vi "Hardware-HHSetup-Host.vi"() -> ()   [LabVIEW 2016]
uses:
  <vilib>/Powertrain Controls/Device Drivers/DCM/HH/RT/Setup.ctl
  <vilib>/Powertrain Controls/Device Drivers/DCM/HH/FPGA/Mode.ctl
  <vilib>/Powertrain Controls/Device Drivers/DCM/Rev0/FPGA/Digital Channel.ctl
  <vilib>/Powertrain Controls/Device Drivers/DCM/HH/RT/Angle Control.ctl
  Shared/Typedefs/HH-Config-Array.ctl
  <vilib>/Powertrain Controls/Device Drivers/DCM/HH/RT/Mode.ctl
  <vilib>/Powertrain Controls/Device Drivers/DCM/HH/RT/ISeq.ctl
  <vilib>/addons/Software Calibration Management/XControls/SubHost.xctl
  <vilib>/Powertrain Controls/Device Drivers/DCM/HH/FPGA/DCM - FPGA - HH.lvlib
  <vilib>/Powertrain Controls/Device Drivers/DCM/HH/RT/DCM - RT - HH.lvlib
  <vilib>/Powertrain Controls/Device Drivers/DCM/Rev0/FPGA/DCM - FPGA.lvlib
  Shared/DSI-Shared.lvlib
panel:
  in  "_Hidden":enum32{"Page 1"}(tab)
  in  "Config":T1=[{"Mode"=enum."Off", "IO Lock State"=FALSE, "Phase 1 FP"=FALSE, "Fault Clear"=FALSE, "ISeq"=[{"Upper [A]"=0.0, "Lower [A]"=0.0, "Duration [s]"=0.0}, {"Upper [A]"=0.0, "Lower [A]"=0.0, "Duration [s]"=0.0}, {"Upper [A]"=0.0, "Lower [A]"=0.0, "Duration [s]"=0.0}, {"Upper [A]"=0.0, "Lower [A]"=0.0, "Duration [s]"=0.0}]}, {"Mode"=enum."Off", "IO Lock State"=FALSE, "Phase 1 FP"=FALSE, "Fault Clear"=FALSE, "ISeq"=[{"Upper [A]"=0.0, "Lower [A]"=0.0, "Duration [s]"=0.0}, {"Upper [A]"=0.0, "Lower [A]"=0.0, "Duration [s]"=0.0}, {"Upper [A]"=0.0, "Lower [A]"=0.0, "Duration [s]"=0.0}, {"Upper [A]"=0.0, "Lower [A]"=0.0, "Duration [s]"=0.0}]}, {"Mode"=enum."Off", "IO Lock State"=FALSE, "Phase 1 FP"=FALSE, "Fault Clear"=FALSE, "ISeq"=[{"Upper [A]"=0.0, "Lower [A]"=0.0, "Duration [s]"=0.0}, {"Upper [A]"=0.0, "Lower [A]"=0.0, "Duration [s]"=0.0}, {"Upper [A]"=0.0, "Lower [A]"=0.0, "Duration [s]"=0.0}, {"Upper [A]"=0.0, "Lower [A]"=0.0, "Duration [s]"=0.0}]}, {"Mode"=enum."Off", "IO Lock State"=FALSE, "Phase 1 FP"=FALSE, "Fault Clear"=FALSE, "ISeq"=[{"Upper [A]"=0.0, "Lower [A]"=0.0, "Duration [s]"=0.0}, {"Upper [A]"=0.0, "Lower [A]"=0.0, "Duration [s]"=0.0}, {"Upper [A]"=0.0, "Lower [A]"=0.0, "Duration [s]"=0.0}, {"Upper [A]"=0.0, "Lower [A]"=0.0, "Duration [s]"=0.0}]}, {"Mode"=enum."Off", "IO Lock State"=FALSE, "Phase 1 FP"=FALSE, "Fault Clear"=FALSE, "ISeq"=[{"Upper [A]"=0.0, "Lower [A]"=0.0, "Duration [s]"=0.0}, {"Upper [A]"=0.0, "Lower [A]"=0.0, "Duration [s]"=0.0}, {"Upper [A]"=0.0, "Lower [A]"=0.0, "Duration [s]"=0.0}, {"Upper [A]"=0.0, "Lower [A]"=0.0, "Duration [s]"=0.0}]}, {"Mode"=enum."Off", "IO Lock State"=FALSE, "Phase 1 FP"=FALSE, "Fault Clear"=FALSE, "ISeq"=[{"Upper [A]"=0.0, "Lower [A]"=0.0, "Duration [s]"=0.0}, {"Upper [A]"=0.0, "Lower [A]"=0.0, "Duration [s]"=0.0}, {"Upper [A]"=0.0, "Lower [A]"=0.0, "Duration [s]"=0.0}, {"Upper [A]"=0.0, "Lower [A]"=0.0, "Duration [s]"=0.0}]}, {"Mode"=enum."Off", "IO Lock State"=FALSE, "Phase 1 FP"=FALSE, "Fault Clear"=FALSE, "ISeq"=[{"Upper [A]"=0.0, "Lower [A]"=0.0, "Duration [s]"=0.0}, {"Upper [A]"=0.0, "Lower [A]"=0.0, "Duration [s]"=0.0}, {"Upper [A]"=0.0, "Lower [A]"=0.0, "Duration [s]"=0.0}, {"Upper [A]"=0.0, "Lower [A]"=0.0, "Duration [s]"=0.0}]}, {"Mode"=enum."Off", "IO Lock State"=FALSE, "Phase 1 FP"=FALSE, "Fault Clear"=FALSE, "ISeq"=[{"Upper [A]"=0.0, "Lower [A]"=0.0, "Duration [s]"=0.0}, {"Upper [A]"=0.0, "Lower [A]"=0.0, "Duration [s]"=0.0}, {"Upper [A]"=0.0, "Lower [A]"=0.0, "Duration [s]"=0.0}, {"Upper [A]"=0.0, "Lower [A]"=0.0, "Duration [s]"=0.0}]}, {"Mode"=enum."Off", "IO Lock State"=FALSE, "Phase 1 FP"=FALSE, "Fault Clear"=FALSE, "ISeq"=[{"Upper [A]"=0.0, "Lower [A]"=0.0, "Duration [s]"=0.0}, {"Upper [A]"=0.0, "Lower [A]"=0.0, "Duration [s]"=0.0}, {"Upper [A]"=0.0, "Lower [A]"=0.0, "Duration [s]"=0.0}, {"Upper [A]"=0.0, "Lower [A]"=0.0, "Duration [s]"=0.0}]}, {"Mode"=enum."Off", "IO Lock State"=FALSE, "Phase 1 FP"=FALSE, "Fault Clear"=FALSE, "ISeq"=[{"Upper [A]"=0.0, "Lower [A]"=0.0, "Duration [s]"=0.0}, {"Upper [A]"=0.0, "Lower [A]"=0.0, "Duration [s]"=0.0}, {"Upper [A]"=0.0, "Lower [A]"=0.0, "Duration [s]"=0.0}, {"Upper [A]"=0.0, "Lower [A]"=0.0, "Duration [s]"=0.0}]}, {"Mode"=enum."Off", "IO Lock State"=FALSE, "Phase 1 FP"=FALSE, "Fault Clear"=FALSE, "ISeq"=[{"Upper [A]"=0.0, "Lower [A]"=0.0, "Duration [s]"=0.0}, {"Upper [A]"=0.0, "Lower [A]"=0.0, "Duration [s]"=0.0}, {"Upper [A]"=0.0, "Lower [A]"=0.0, "Duration [s]"=0.0}, {"Upper [A]"=0.0, "Lower [A]"=0.0, "Duration [s]"=0.0}]}, {"Mode"=enum."Off", "IO Lock State"=FALSE, "Phase 1 FP"=FALSE, "Fault Clear"=FALSE, "ISeq"=[{"Upper [A]"=0.0, "Lower [A]"=0.0, "Duration [s]"=0.0}, {"Upper [A]"=0.0, "Lower [A]"=0.0, "Duration [s]"=0.0}, {"Upper [A]"=0.0, "Lower [A]"=0.0, "Duration [s]"=0.0}, {"Upper [A]"=0.0, "Lower [A]"=0.0, "Duration [s]"=0.0}]}] {"ISeq"."Duration [s]" min=0 max=26 format="%#_3p"; "ISeq"."Lower [A]" min=0 max=8 format="%#_3p"; "ISeq"."Upper [A]" min=0 max=8 format="%#_3p"}
  in  "Cmd":T4[](array[typedef])=[{"Mode"=enum."Off", "Digital Input"=enum."Unused", "Polarity"=FALSE, "Frequency [Hz]"=0.0, "Duty Cycle [%]"=0.0, "TDC Offset [CAD]"=0.0, "Window Start [DBTDC]"=0.0, "Window End [DBTDC]"=0.0, "Angles"=[{"Enable"=FALSE, "Location [DBTDC]"=0.0, "Duration [s]"=0.0}, {"Enable"=FALSE, "Location [DBTDC]"=0.0, "Duration [s]"=0.0}, {"Enable"=FALSE, "Location [DBTDC]"=0.0, "Duration [s]"=0.0}, {"Enable"=FALSE, "Location [DBTDC]"=0.0, "Duration [s]"=0.0}], "Skip Fire"=FALSE, "Skip Fire Index"=0}, {"Mode"=enum."Off", "Digital Input"=enum."Unused", "Polarity"=FALSE, "Frequency [Hz]"=0.0, "Duty Cycle [%]"=0.0, "TDC Offset [CAD]"=0.0, "Window Start [DBTDC]"=0.0, "Window End [DBTDC]"=0.0, "Angles"=[{"Enable"=FALSE, "Location [DBTDC]"=0.0, "Duration [s]"=0.0}, {"Enable"=FALSE, "Location [DBTDC]"=0.0, "Duration [s]"=0.0}, {"Enable"=FALSE, "Location [DBTDC]"=0.0, "Duration [s]"=0.0}, {"Enable"=FALSE, "Location [DBTDC]"=0.0, "Duration [s]"=0.0}], "Skip Fire"=FALSE, "Skip Fire Index"=0}, {"Mode"=enum."Off", "Digital Input"=enum."Unused", "Polarity"=FALSE, "Frequency [Hz]"=0.0, "Duty Cycle [%]"=0.0, "TDC Offset [CAD]"=0.0, "Window Start [DBTDC]"=0.0, "Window End [DBTDC]"=0.0, "Angles"=[{"Enable"=FALSE, "Location [DBTDC]"=0.0, "Duration [s]"=0.0}, {"Enable"=FALSE, "Location [DBTDC]"=0.0, "Duration [s]"=0.0}, {"Enable"=FALSE, "Location [DBTDC]"=0.0, "Duration [s]"=0.0}, {"Enable"=FALSE, "Location [DBTDC]"=0.0, "Duration [s]"=0.0}], "Skip Fire"=FALSE, "Skip Fire Index"=0}, {"Mode"=enum."Off", "Digital Input"=enum."Unused", "Polarity"=FALSE, "Frequency [Hz]"=0.0, "Duty Cycle [%]"=0.0, "TDC Offset [CAD]"=0.0, "Window Start [DBTDC]"=0.0, "Window End [DBTDC]"=0.0, "Angles"=[{"Enable"=FALSE, "Location [DBTDC]"=0.0, "Duration [s]"=0.0}, {"Enable"=FALSE, "Location [DBTDC]"=0.0, "Duration [s]"=0.0}, {"Enable"=FALSE, "Location [DBTDC]"=0.0, "Duration [s]"=0.0}, {"Enable"=FALSE, "Location [DBTDC]"=0.0, "Duration [s]"=0.0}], "Skip Fire"=FALSE, "Skip Fire Index"=0}, {"Mode"=enum."Off", "Digital Input"=enum."Unused", "Polarity"=FALSE, "Frequency [Hz]"=0.0, "Duty Cycle [%]"=0.0, "TDC Offset [CAD]"=0.0, "Window Start [DBTDC]"=0.0, "Window End [DBTDC]"=0.0, "Angles"=[{"Enable"=FALSE, "Location [DBTDC]"=0.0, "Duration [s]"=0.0}, {"Enable"=FALSE, "Location [DBTDC]"=0.0, "Duration [s]"=0.0}, {"Enable"=FALSE, "Location [DBTDC]"=0.0, "Duration [s]"=0.0}, {"Enable"=FALSE, "Location [DBTDC]"=0.0, "Duration [s]"=0.0}], "Skip Fire"=FALSE, "Skip Fire Index"=0}, {"Mode"=enum."Off", "Digital Input"=enum."Unused", "Polarity"=FALSE, "Frequency [Hz]"=0.0, "Duty Cycle [%]"=0.0, "TDC Offset [CAD]"=0.0, "Window Start [DBTDC]"=0.0, "Window End [DBTDC]"=0.0, "Angles"=[{"Enable"=FALSE, "Location [DBTDC]"=0.0, "Duration [s]"=0.0}, {"Enable"=FALSE, "Location [DBTDC]"=0.0, "Duration [s]"=0.0}, {"Enable"=FALSE, "Location [DBTDC]"=0.0, "Duration [s]"=0.0}, {"Enable"=FALSE, "Location [DBTDC]"=0.0, "Duration [s]"=0.0}], "Skip Fire"=FALSE, "Skip Fire Index"=0}, {"Mode"=enum."Off", "Digital Input"=enum."Unused", "Polarity"=FALSE, "Frequency [Hz]"=0.0, "Duty Cycle [%]"=0.0, "TDC Offset [CAD]"=0.0, "Window Start [DBTDC]"=0.0, "Window End [DBTDC]"=0.0, "Angles"=[{"Enable"=FALSE, "Location [DBTDC]"=0.0, "Duration [s]"=0.0}, {"Enable"=FALSE, "Location [DBTDC]"=0.0, "Duration [s]"=0.0}, {"Enable"=FALSE, "Location [DBTDC]"=0.0, "Duration [s]"=0.0}, {"Enable"=FALSE, "Location [DBTDC]"=0.0, "Duration [s]"=0.0}], "Skip Fire"=FALSE, "Skip Fire Index"=0}, {"Mode"=enum."Off", "Digital Input"=enum."Unused", "Polarity"=FALSE, "Frequency [Hz]"=0.0, "Duty Cycle [%]"=0.0, "TDC Offset [CAD]"=0.0, "Window Start [DBTDC]"=0.0, "Window End [DBTDC]"=0.0, "Angles"=[{"Enable"=FALSE, "Location [DBTDC]"=0.0, "Duration [s]"=0.0}, {"Enable"=FALSE, "Location [DBTDC]"=0.0, "Duration [s]"=0.0}, {"Enable"=FALSE, "Location [DBTDC]"=0.0, "Duration [s]"=0.0}, {"Enable"=FALSE, "Location [DBTDC]"=0.0, "Duration [s]"=0.0}], "Skip Fire"=FALSE, "Skip Fire Index"=0}, {"Mode"=enum."Off", "Digital Input"=enum."Unused", "Polarity"=FALSE, "Frequency [Hz]"=0.0, "Duty Cycle [%]"=0.0, "TDC Offset [CAD]"=0.0, "Window Start [DBTDC]"=0.0, "Window End [DBTDC]"=0.0, "Angles"=[{"Enable"=FALSE, "Location [DBTDC]"=0.0, "Duration [s]"=0.0}, {"Enable"=FALSE, "Location [DBTDC]"=0.0, "Duration [s]"=0.0}, {"Enable"=FALSE, "Location [DBTDC]"=0.0, "Duration [s]"=0.0}, {"Enable"=FALSE, "Location [DBTDC]"=0.0, "Duration [s]"=0.0}], "Skip Fire"=FALSE, "Skip Fire Index"=0}, {"Mode"=enum."Off", "Digital Input"=enum."Unused", "Polarity"=FALSE, "Frequency [Hz]"=0.0, "Duty Cycle [%]"=0.0, "TDC Offset [CAD]"=0.0, "Window Start [DBTDC]"=0.0, "Window End [DBTDC]"=0.0, "Angles"=[{"Enable"=FALSE, "Location [DBTDC]"=0.0, "Duration [s]"=0.0}, {"Enable"=FALSE, "Location [DBTDC]"=0.0, "Duration [s]"=0.0}, {"Enable"=FALSE, "Location [DBTDC]"=0.0, "Duration [s]"=0.0}, {"Enable"=FALSE, "Location [DBTDC]"=0.0, "Duration [s]"=0.0}], "Skip Fire"=FALSE, "Skip Fire Index"=0}, {"Mode"=enum."Off", "Digital Input"=enum."Unused", "Polarity"=FALSE, "Frequency [Hz]"=0.0, "Duty Cycle [%]"=0.0, "TDC Offset [CAD]"=0.0, "Window Start [DBTDC]"=0.0, "Window End [DBTDC]"=0.0, "Angles"=[{"Enable"=FALSE, "Location [DBTDC]"=0.0, "Duration [s]"=0.0}, {"Enable"=FALSE, "Location [DBTDC]"=0.0, "Duration [s]"=0.0}, {"Enable"=FALSE, "Location [DBTDC]"=0.0, "Duration [s]"=0.0}, {"Enable"=FALSE, "Location [DBTDC]"=0.0, "Duration [s]"=0.0}], "Skip Fire"=FALSE, "Skip Fire Index"=0}, {"Mode"=enum."Off", "Digital Input"=enum."Unused", "Polarity"=FALSE, "Frequency [Hz]"=0.0, "Duty Cycle [%]"=0.0, "TDC Offset [CAD]"=0.0, "Window Start [DBTDC]"=0.0, "Window End [DBTDC]"=0.0, "Angles"=[{"Enable"=FALSE, "Location [DBTDC]"=0.0, "Duration [s]"=0.0}, {"Enable"=FALSE, "Location [DBTDC]"=0.0, "Duration [s]"=0.0}, {"Enable"=FALSE, "Location [DBTDC]"=0.0, "Duration [s]"=0.0}, {"Enable"=FALSE, "Location [DBTDC]"=0.0, "Duration [s]"=0.0}], "Skip Fire"=FALSE, "Skip Fire Index"=0}] {"Skip Fire Index" max=7; "Angles"."Duration [s]" format="%#_3p"; "Frequency [Hz]" format="%#_3p"}
  in  "_Refresh":bool
  in  "AdaptMode":u32
  in  "ChannelNames":string[](array[string])
  out "_Disabled Configs":i32[](array[numeric])
  in  "Scope":T8(xcontrol)
  in  "_Config Tab":enum32{"Page 1"}(tab)
  in  "_Cmd Tab":enum32{"Page 1"}(tab)
  in  "_Icon tabs":enum32{"Off", "Lo", "Hi", "PFI", "FullH"}(tab)
  in  "Status":T8(xcontrol)
  in  "_AdaptMode":bool caption="Adapt Mode"
  in  "_Channel Name":string caption="Channel Name"
  in  "_Command Element":T4={"Mode"=enum."Off", "Digital Input"=enum."Unused", "Polarity"=FALSE, "Frequency [Hz]"=0.0, "Duty Cycle [%]"=0.0, "TDC Offset [CAD]"=0.0, "Window Start [DBTDC]"=0.0, "Window End [DBTDC]"=0.0, "Angles"=[{"Enable"=FALSE, "Location [DBTDC]"=0.0, "Duration [s]"=0.0}, {"Enable"=FALSE, "Location [DBTDC]"=0.0, "Duration [s]"=0.0}, {"Enable"=FALSE, "Location [DBTDC]"=0.0, "Duration [s]"=0.0}, {"Enable"=FALSE, "Location [DBTDC]"=0.0, "Duration [s]"=0.0}], "Skip Fire"=FALSE, "Skip Fire Index"=0} caption="Command Setup" {"Skip Fire Index" max=7; "Angles"."Duration [s]" format="%#_3p"; "Frequency [Hz]" format="%#_3p"}
  in  "_Config Element":T9={"Mode"=enum."Off", "IO Lock State"=FALSE, "Phase 1 FP"=FALSE, "Fault Clear"=FALSE, "ISeq"=[{"Upper [A]"=0.0, "Lower [A]"=0.0, "Duration [s]"=0.0}, {"Upper [A]"=0.0, "Lower [A]"=0.0, "Duration [s]"=0.0}, {"Upper [A]"=0.0, "Lower [A]"=0.0, "Duration [s]"=0.0}, {"Upper [A]"=0.0, "Lower [A]"=0.0, "Duration [s]"=0.0}]} caption="Channel Configuration" {"ISeq"."Duration [s]" min=0 max=26 format="%#_3p"; "ISeq"."Lower [A]" min=0 max=8 format="%#_3p"; "ISeq"."Upper [A]" min=0 max=8 format="%#_3p"}
  in  "_HH Channels":i32[](listbox) caption="Half-H Channel Summary"
  # "Half-H Drive Setup & Control"
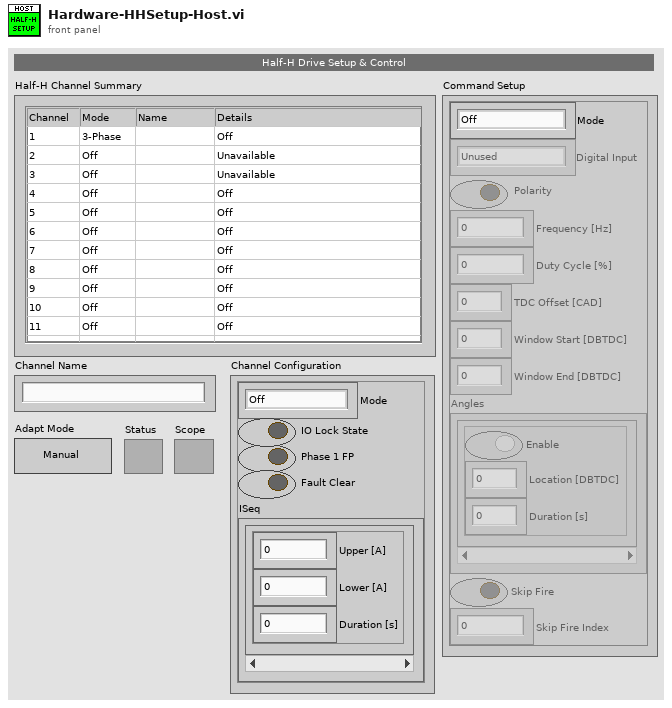
[diagram p1: front panel]
types:
  T1 = typedef "DSI-Shared.lvlib/HH-Config-Array.ctl" = cluster{"Mode":T2, "IO Lock State":bool, "Phase 1 FP":bool, "Fault Clear":bool, "ISeq":T3[]}[]
  T2 = typedef "DCM - RT - HH.lvlib/Mode.ctl" = enum16{"Off", "Lowside", "Highside", "PFI", "Full H", "3-Phase"}
  T3 = typedef "DCM - RT - HH.lvlib/ISeq.ctl" = cluster{"Upper [A]":sgl, "Lower [A]":sgl, "Duration [s]":sgl}
  T4 = typedef "DCM - RT - HH.lvlib/Setup.ctl" = cluster{"Mode":T5, "Digital Input":T6, "Polarity":bool, "Frequency [Hz]":sgl, "Duty Cycle [%]":sgl, "TDC Offset [CAD]":sgl, "Window Start [DBTDC]":sgl, "Window End [DBTDC]":sgl, "Angles":T7[], "Skip Fire":bool, "Skip Fire Index":u8}
  T5 = typedef "DCM - FPGA - HH.lvlib/Mode.ctl" = enum8{"Off", "Direct", "Pulse Width Modulation", "Engine Position Tracking"}
  T6 = typedef "DCM - FPGA.lvlib/Digital Channel.ctl" = enum8{"Unused", "User OS", "Diff IO 1", "Diff IO 2", "Diff IO 3", "Diff IO 4", "Diff IO 5", "Diff IO 6", "Diff IO 7", "Diff IO 8", "Aux 1", "Aux 2", "Aux 3", "Aux 4", "Aux 5", "Aux 6", "Aux 7", "Aux 8", "Aux 9", "Aux 10", "Aux 11", "Aux 12", "Aux 13", "Aux 14", "Aux 15", "Aux 16"}
  T7 = typedef "DCM - RT - HH.lvlib/Angle Control.ctl" = cluster{"Enable":bool, "Location [DBTDC]":sgl, "Duration [s]":sgl}
  T8 = cluster{"Name":string, "Host VI":path, "Pairing File":path, "Display Name":string}
  T9 = cluster{"Mode":T2, "IO Lock State":bool, "Phase 1 FP":bool, "Fault Clear":bool, "ISeq":T3[]}
  T10 = enum8{"Enabled", "Disabled", "Disabled and Grayed Out"}
  T11 = typedef "DCM - RT - HH.lvlib/Config.ctl" = cluster{"Mode":T2, "IO Lock State":bool, "Phase 1 FP":bool, "Fault Clear":bool, "ISeq":T3[]}
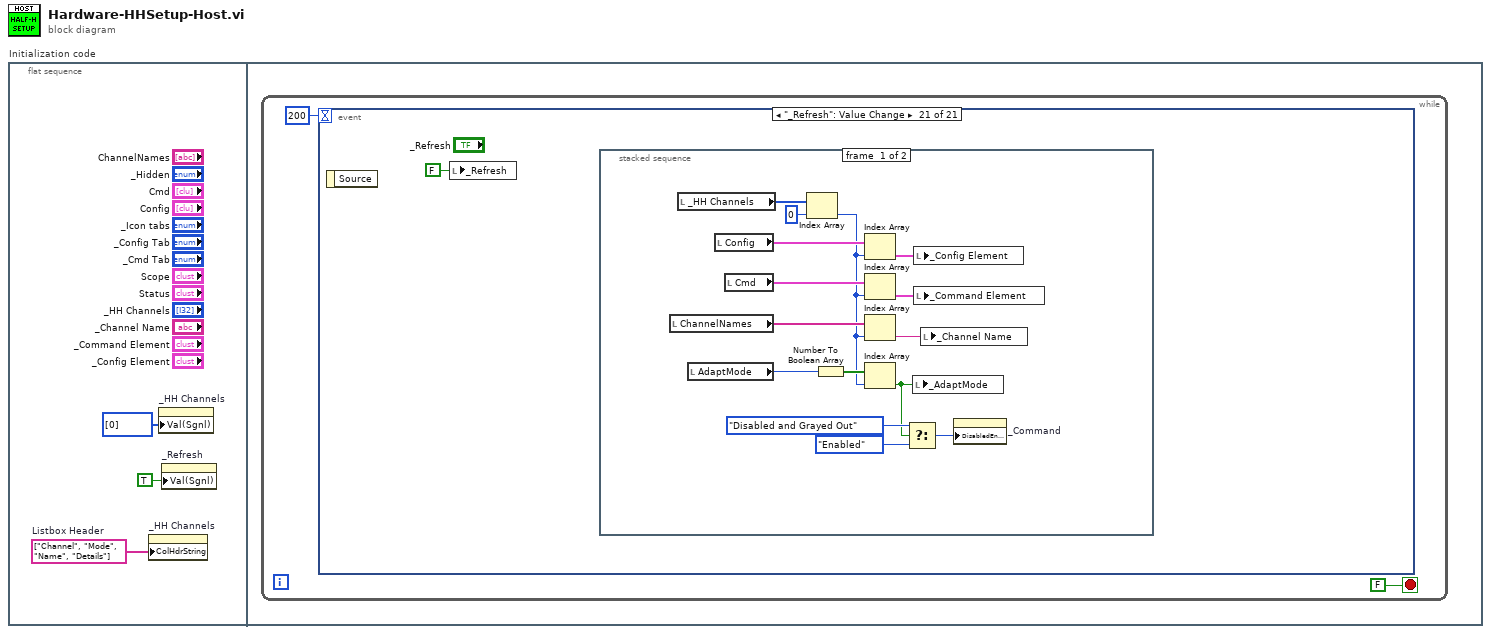
[diagram p0: block diagram]
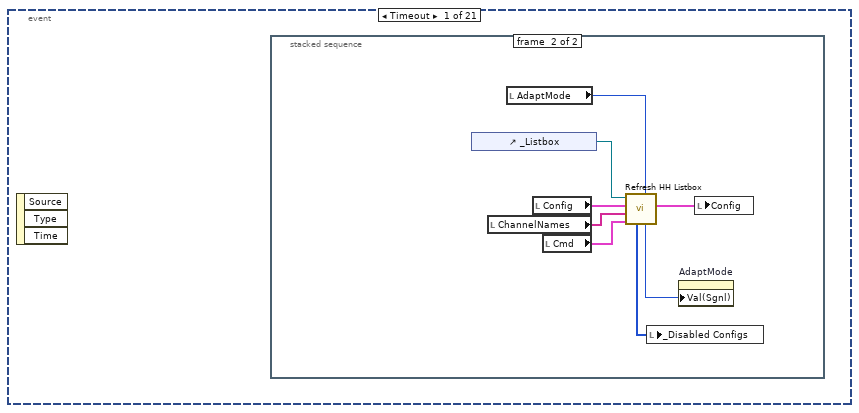
[diagram p2: hidden frame]
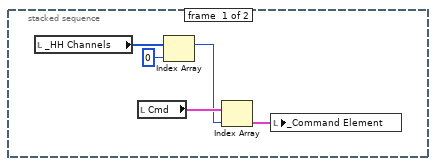
[diagram p3: hidden frame]
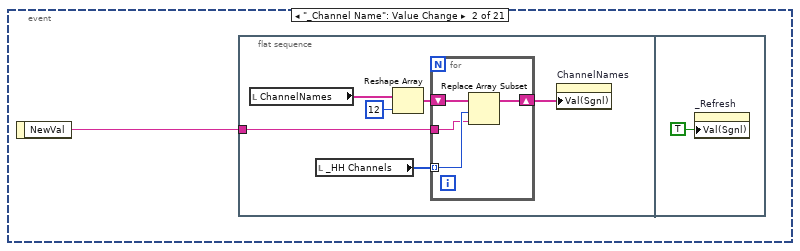
[diagram p4: hidden frame]
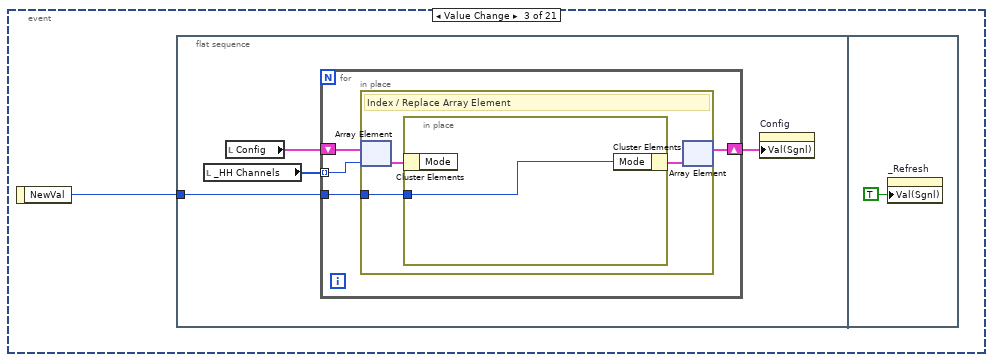
[diagram p5: hidden frame]
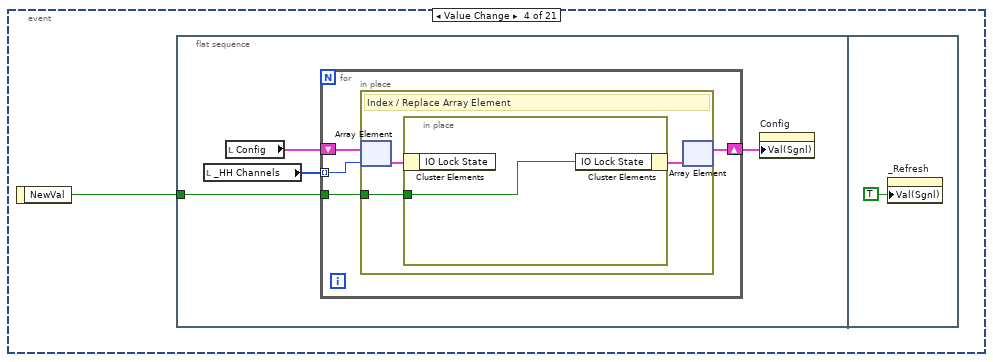
[diagram p6: hidden frame]
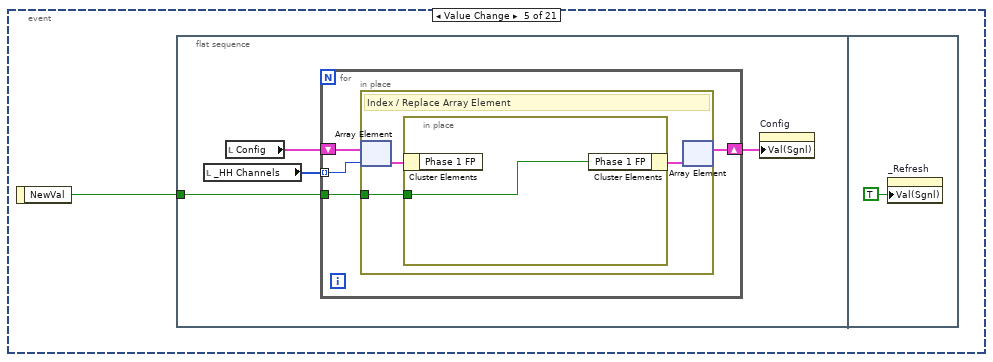
[diagram p7: hidden frame]
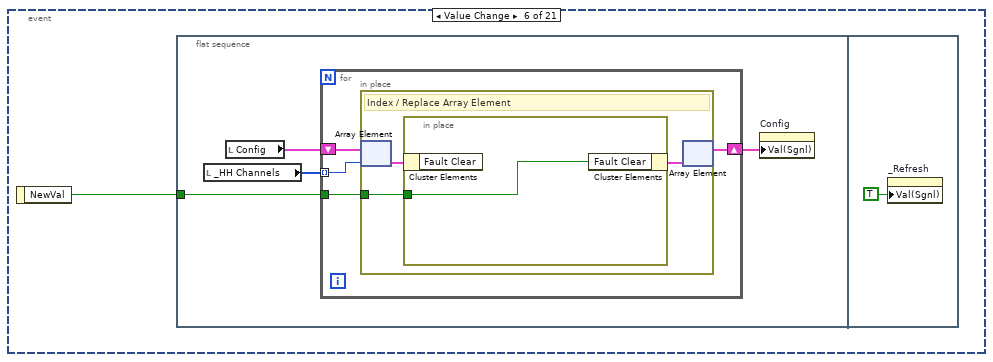
[diagram p8: hidden frame]
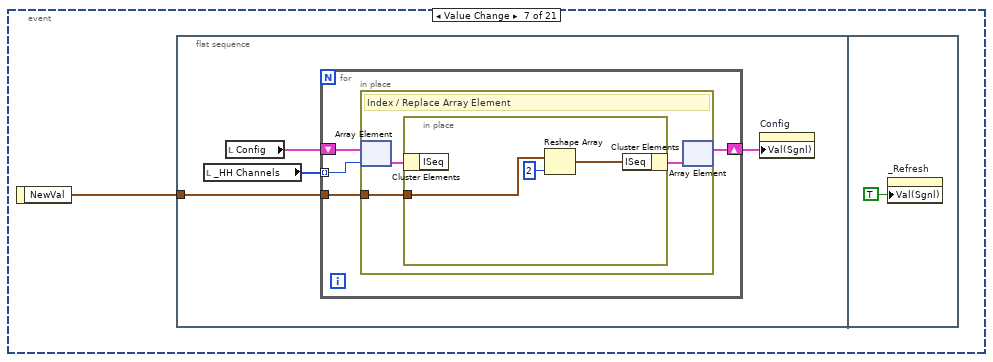
[diagram p9: hidden frame]
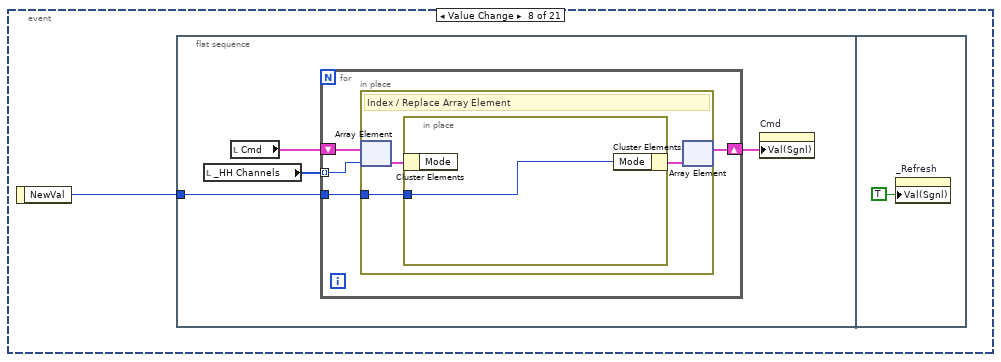
[diagram p10: hidden frame]
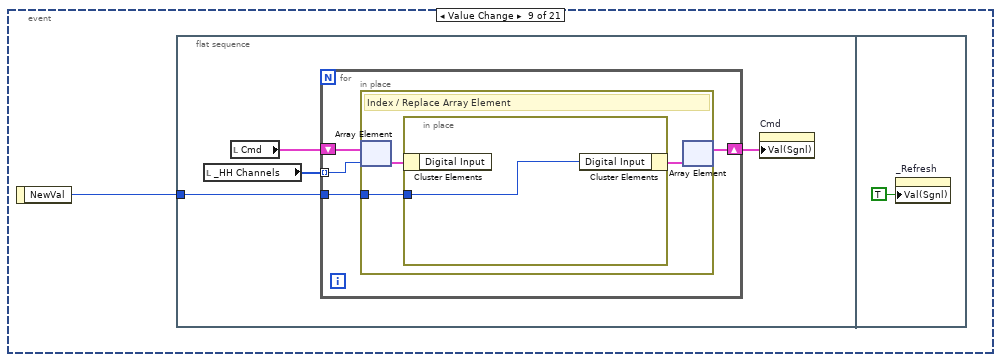
[diagram p11: hidden frame]
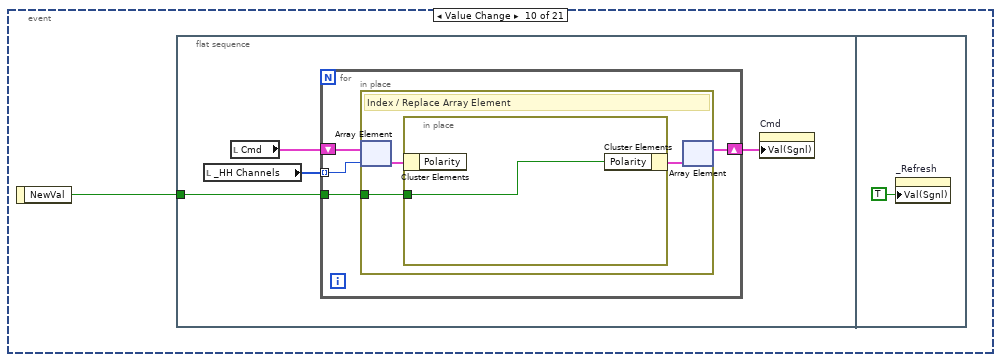
[diagram p12: hidden frame]
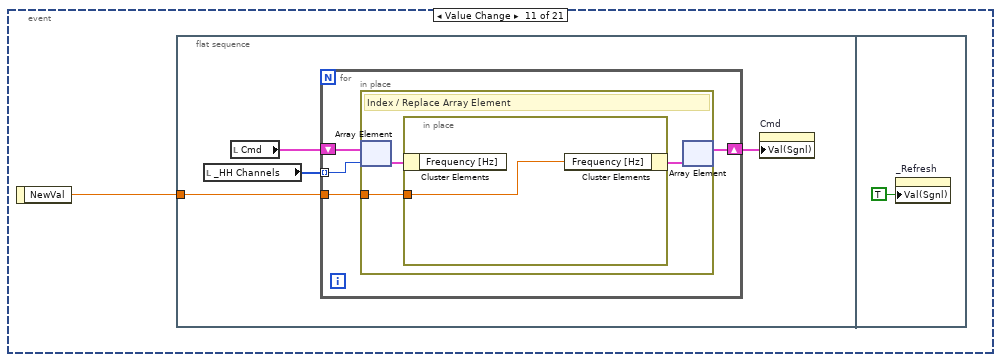
[diagram p13: hidden frame]
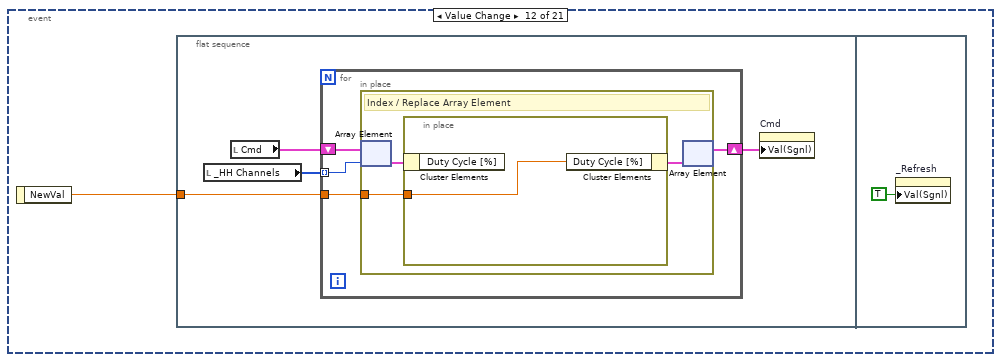
[diagram p14: hidden frame]
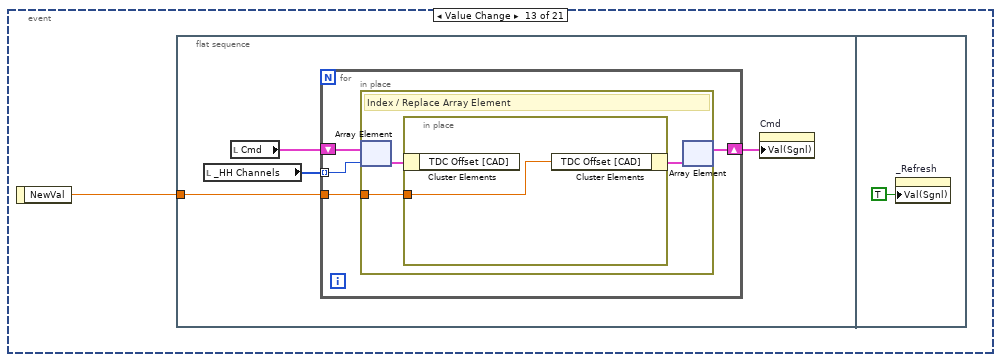
[diagram p15: hidden frame]
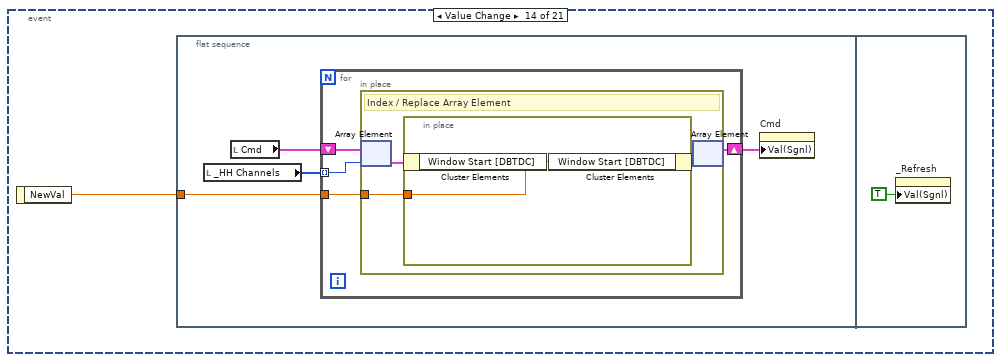
[diagram p16: hidden frame]
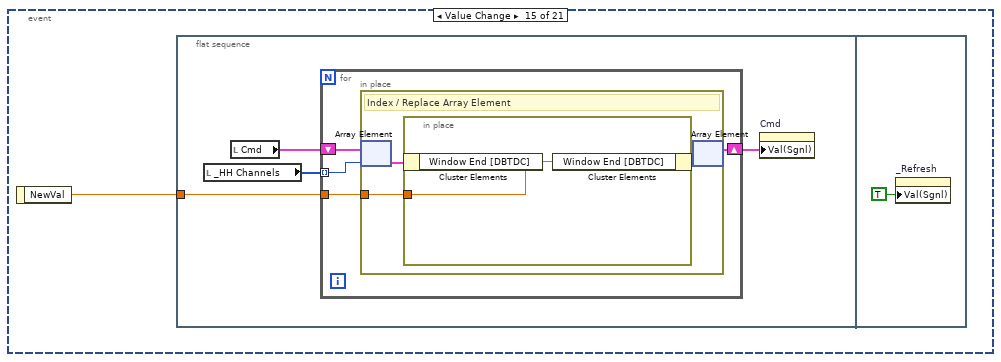
[diagram p17: hidden frame]
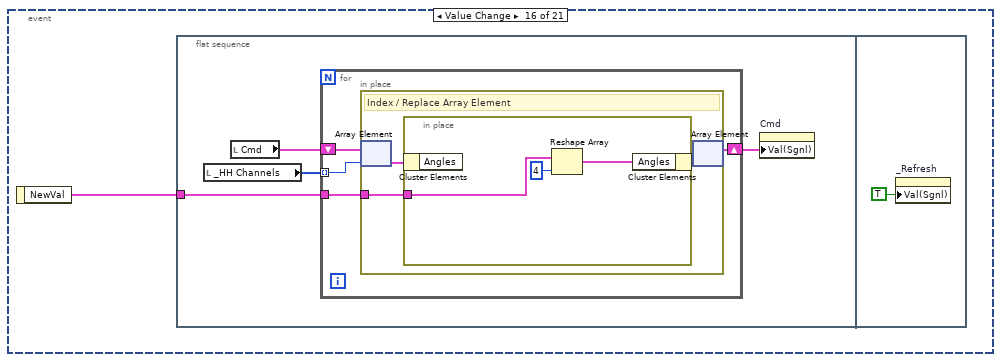
[diagram p18: hidden frame]
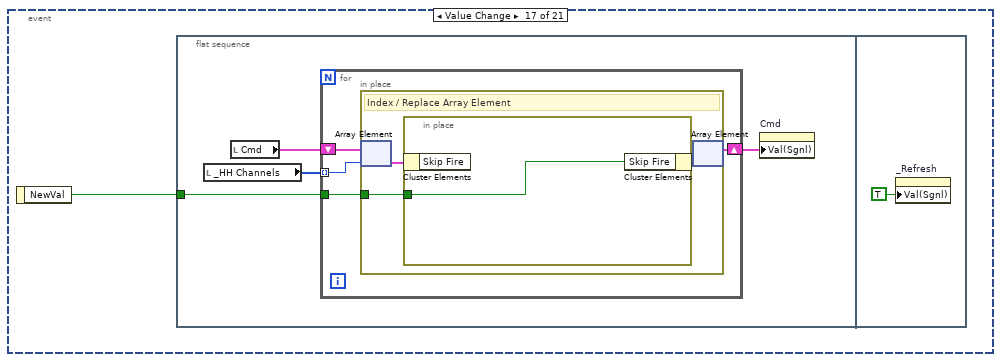
[diagram p19: hidden frame]
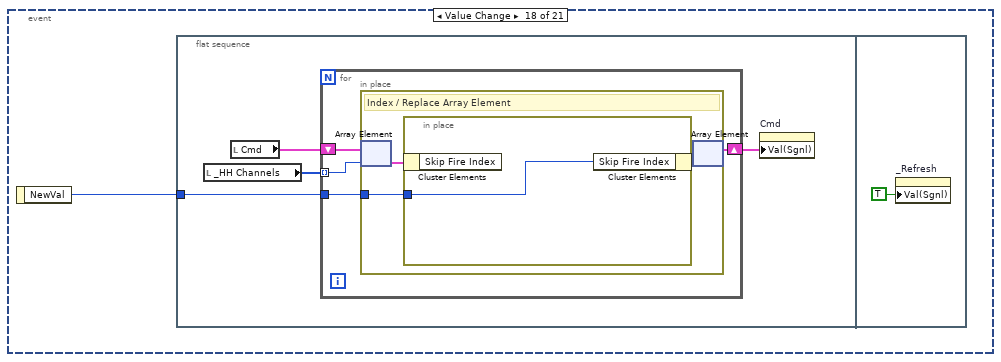
[diagram p20: hidden frame]
diagram:
  n1 = flat-sequence "Initialization code" {
    frame #0 {
      w1 = string[] ["Channel", "Mode", "Name", "Details"]  # Listbox Header
      n2 = property on="_HH Channels" class="MCListbox (strict)"("ColHdrString"=w1) -> ()  [unwired: 2 in, 2 out]
      n3 = property on="_HH Channels" class="MCListbox (strict)"("Val(Sgnl)"=i32[] [0] ("Value (Signaling)")) -> ()  [unwired: 2 in, 2 out]
      n4 = property on="_Refresh" class="Bool (strict)"("Val(Sgnl)"=TRUE ("Value (Signaling)")) -> ()  [unwired: 2 in, 2 out]
    }
    frame #1 {
      n5 = while {
        stop <- FALSE stop-if-true
        n6 = event shown="[20] \"_Refresh\": Value Change" {
          selector: _ -> [_ _ _ _ _ _ _ _ _ _ _ _ _ _ _ _ _ _ _ _ _]
          dyn-events: _ -> [_ _ _ _ _ _ _ _ _ _ _ _ _ _ _ _ _ _ _ _ _]
          timeout: 200 -> [_ _ _ _ _ _ _ _ _ _ _ _ _ _ _ _ _ _ _ _ _]
          event Timeout {
            n7 = event-data() -> ()  [unwired: 4 out]
            n8 = stacked-sequence {
              frame #0 {
                n9 = local read "_HH Channels"() -> (w10:i32[])
                n10 = local read "Cmd"() -> (w9:T4[])
                n11 = Index Array(array=w10, index=0) -> (element=w8:i32)
                n12 = Index Array(array=w9, index=w8) -> (element=w6:T4)
                n13 = local write "_Command Element"(w6) -> ()
              }
              frame #1 {
                n14 = control-ref of="_Listbox"() -> (w13:refnum<vi>)
                n15 = local read "ChannelNames"() -> (w11:string[])
                n16 = local read "AdaptMode"() -> (w16:u32)
                n17 = local read "Config"() -> (w18:T1)
                n18 = local read "Cmd"() -> (w17:T4[])
                n19 = call "Refresh HH Listbox.vi"("AdaptMode"=w16, "Command"=w17, "Names"=w11, "Config"=w18, "_Listbox"=w13) -> ("Config out"=w14:T11[], "AdaptMode"=w15:u32, "Disabled Configs"=w12:i32[])  [unwired: 3 in, 1 out]
                n20 = local write "_Disabled Configs"(w12) -> ()
                n21 = property on="AdaptMode" class="DigNum (strict)"("Val(Sgnl)"=w15) -> ()  [unwired: 2 in, 2 out]
                n22 = local write "Config"(w14) -> ()
              }
            }
          }
          event "_Channel Name": Value Change {
            n23 = event-data() -> ("NewVal"=w19:string)  [unwired: 1 out]
            n24 = flat-sequence {
              tunnel: w19 -> [w22]
              frame #0 {
                n25 = local read "ChannelNames"() -> (w21:string[])
                n26 = local read "_HH Channels"() -> (w25:i32[])
                n27 = Reshape Array(w21, 12 ("dimension size")) -> (w23:string[])
                n28 = for {
                  tunnel: w25 -> [w27] mode=indexing
                  shift-right: [w28] -> w20
                  shift-left: w23 -> [w29]
                  tunnel: w22 -> [w26]
                  n29 = Replace Array Subset(array=w29, new element=w26, index=w27) -> (w28:string[])
                }
                n30 = property on="ChannelNames" class="Arr (strict)"("Val(Sgnl)"=w20) -> ()  [unwired: 2 in, 2 out]
              }
              frame #1 {
                n31 = property on="_Refresh" class="Bool (strict)"("Val(Sgnl)"=TRUE ("Value (Signaling)")) -> ()  [unwired: 2 in, 2 out]
              }
            }
          }
          event Value Change {
            n32 = event-data() -> ("NewVal"=w31:T2)  [unwired: 1 out]
            n33 = flat-sequence {
              tunnel: w31 -> [w34]
              frame #0 {
                n34 = local read "_HH Channels"() -> (w35:i32[])
                n35 = local read "Config"() -> (w33:T1)
                n36 = for {
                  tunnel: w35 -> [w38] mode=indexing
                  shift-right: [w37] -> w32
                  shift-left: w33 -> [w39]
                  tunnel: w34 -> [w36]
                  n37 = in-place {
                    in-place-border: w36 -> [w40]
                    # "Index / Replace Array Element"
                    n38 = in-place-array #1(w39, w38) -> (w42:T9)
                    n39 = in-place {
                      in-place-border: w40 -> [w43]
                      n40 = in-place-cluster #2(w42) -> ()  [unwired: 1 out]
                      n41 = in-place-cluster #2("Mode"=w43) -> (w41:T9)
                    }
                    n42 = in-place-array #1(w41) -> (w37:T1)  [unwired: 1 out]
                  }
                }
                n43 = property on="Config" class="Arr (strict)"("Val(Sgnl)"=w32) -> ()  [unwired: 2 in, 2 out]
              }
              frame #1 {
                n44 = property on="_Refresh" class="Bool (strict)"("Val(Sgnl)"=TRUE ("Value (Signaling)")) -> ()  [unwired: 2 in, 2 out]
              }
            }
          }
          event "_Config Element.IO Lock State": Value Change {
            n45 = event-data() -> ("NewVal"=w45:bool)  [unwired: 1 out]
            n46 = flat-sequence {
              tunnel: w45 -> [w48]
              frame #0 {
                n47 = local read "_HH Channels"() -> (w49:i32[])
                n48 = local read "Config"() -> (w47:T1)
                n49 = for {
                  tunnel: w49 -> [w52] mode=indexing
                  shift-right: [w51] -> w46
                  shift-left: w47 -> [w53]
                  tunnel: w48 -> [w50]
                  n50 = in-place {
                    in-place-border: w50 -> [w54]
                    # "Index / Replace Array Element"
                    n51 = in-place-array #3(w53, w52) -> (w56:T9)
                    n52 = in-place {
                      in-place-border: w54 -> [w57]
                      n53 = in-place-cluster #4(w56) -> ()  [unwired: 1 out]
                      n54 = in-place-cluster #4("IO Lock State"=w57) -> (w55:T9)
                    }
                    n55 = in-place-array #3(w55) -> (w51:T1)  [unwired: 1 out]
                  }
                }
                n56 = property on="Config" class="Arr (strict)"("Val(Sgnl)"=w46) -> ()  [unwired: 2 in, 2 out]
              }
              frame #1 {
                n57 = property on="_Refresh" class="Bool (strict)"("Val(Sgnl)"=TRUE ("Value (Signaling)")) -> ()  [unwired: 2 in, 2 out]
              }
            }
          }
          event "_Config Element.Phase 1 FP": Value Change {
            n58 = event-data() -> ("NewVal"=w59:bool)  [unwired: 1 out]
            n59 = flat-sequence {
              tunnel: w59 -> [w62]
              frame #0 {
                n60 = local read "_HH Channels"() -> (w63:i32[])
                n61 = local read "Config"() -> (w61:T1)
                n62 = for {
                  tunnel: w63 -> [w66] mode=indexing
                  shift-right: [w65] -> w60
                  shift-left: w61 -> [w67]
                  tunnel: w62 -> [w64]
                  n63 = in-place {
                    in-place-border: w64 -> [w68]
                    # "Index / Replace Array Element"
                    n64 = in-place-array #5(w67, w66) -> (w70:T9)
                    n65 = in-place {
                      in-place-border: w68 -> [w71]
                      n66 = in-place-cluster #6(w70) -> ()  [unwired: 1 out]
                      n67 = in-place-cluster #6("Phase 1 FP"=w71) -> (w69:T9)
                    }
                    n68 = in-place-array #5(w69) -> (w65:T1)  [unwired: 1 out]
                  }
                }
                n69 = property on="Config" class="Arr (strict)"("Val(Sgnl)"=w60) -> ()  [unwired: 2 in, 2 out]
              }
              frame #1 {
                n70 = property on="_Refresh" class="Bool (strict)"("Val(Sgnl)"=TRUE ("Value (Signaling)")) -> ()  [unwired: 2 in, 2 out]
              }
            }
          }
          event "_Config Element.Fault Clear": Value Change {
            n71 = event-data() -> ("NewVal"=w73:bool)  [unwired: 1 out]
            n72 = flat-sequence {
              tunnel: w73 -> [w76]
              frame #0 {
                n73 = local read "_HH Channels"() -> (w77:i32[])
                n74 = local read "Config"() -> (w75:T1)
                n75 = for {
                  tunnel: w77 -> [w80] mode=indexing
                  shift-right: [w79] -> w74
                  shift-left: w75 -> [w81]
                  tunnel: w76 -> [w78]
                  n76 = in-place {
                    in-place-border: w78 -> [w82]
                    # "Index / Replace Array Element"
                    n77 = in-place-array #7(w81, w80) -> (w84:T9)
                    n78 = in-place {
                      in-place-border: w82 -> [w85]
                      n79 = in-place-cluster #8(w84) -> ()  [unwired: 1 out]
                      n80 = in-place-cluster #8("Fault Clear"=w85) -> (w83:T9)
                    }
                    n81 = in-place-array #7(w83) -> (w79:T1)  [unwired: 1 out]
                  }
                }
                n82 = property on="Config" class="Arr (strict)"("Val(Sgnl)"=w74) -> ()  [unwired: 2 in, 2 out]
              }
              frame #1 {
                n83 = property on="_Refresh" class="Bool (strict)"("Val(Sgnl)"=TRUE ("Value (Signaling)")) -> ()  [unwired: 2 in, 2 out]
              }
            }
          }
          event "_Config Element.ISeq": Value Change {
            n84 = event-data() -> ("NewVal"=w87:T3[])  [unwired: 1 out]
            n85 = flat-sequence {
              tunnel: w87 -> [w90]
              frame #0 {
                n86 = local read "_HH Channels"() -> (w91:i32[])
                n87 = local read "Config"() -> (w89:T1)
                n88 = for {
                  tunnel: w91 -> [w94] mode=indexing
                  shift-right: [w93] -> w88
                  shift-left: w89 -> [w95]
                  tunnel: w90 -> [w92]
                  n89 = in-place {
                    in-place-border: w92 -> [w96]
                    # "Index / Replace Array Element"
                    n90 = in-place-array #9(w95, w94) -> (w98:T9)
                    n91 = in-place {
                      in-place-border: w96 -> [w100]
                      n92 = in-place-cluster #10(w98) -> ()  [unwired: 1 out]
                      n93 = Reshape Array(w100, 2 ("dimension size")) -> (w99:T3[])
                      n94 = in-place-cluster #10("ISeq"=w99) -> (w97:T9)
                    }
                    n95 = in-place-array #9(w97) -> (w93:T1)  [unwired: 1 out]
                  }
                }
                n96 = property on="Config" class="Arr (strict)"("Val(Sgnl)"=w88) -> ()  [unwired: 2 in, 2 out]
              }
              frame #1 {
                n97 = property on="_Refresh" class="Bool (strict)"("Val(Sgnl)"=TRUE ("Value (Signaling)")) -> ()  [unwired: 2 in, 2 out]
              }
            }
          }
          event Value Change {
            n98 = event-data() -> ("NewVal"=w103:T5)  [unwired: 1 out]
            n99 = flat-sequence {
              tunnel: w103 -> [w106]
              frame #0 {
                n100 = local read "_HH Channels"() -> (w107:i32[])
                n101 = local read "Cmd"() -> (w105:T4[])
                n102 = for {
                  tunnel: w107 -> [w110] mode=indexing
                  shift-right: [w109] -> w104
                  shift-left: w105 -> [w111]
                  tunnel: w106 -> [w108]
                  n103 = in-place {
                    in-place-border: w108 -> [w112]
                    # "Index / Replace Array Element"
                    n104 = in-place-array #11(w111, w110) -> (w114:T4)
                    n105 = in-place {
                      in-place-border: w112 -> [w115]
                      n106 = in-place-cluster #12(w114) -> ()  [unwired: 1 out]
                      n107 = in-place-cluster #12("Mode"=w115) -> (w113:T4)
                    }
                    n108 = in-place-array #11(w113) -> (w109:T4[])  [unwired: 1 out]
                  }
                }
                n109 = property on="Cmd" class="Arr (strict)"("Val(Sgnl)"=w104) -> ()  [unwired: 2 in, 2 out]
              }
              frame #1 {
                n110 = property on="_Refresh" class="Bool (strict)"("Val(Sgnl)"=TRUE ("Value (Signaling)")) -> ()  [unwired: 2 in, 2 out]
              }
            }
          }
          event Value Change {
            n111 = event-data() -> ("NewVal"=w117:T6)  [unwired: 1 out]
            n112 = flat-sequence {
              tunnel: w117 -> [w120]
              frame #0 {
                n113 = local read "_HH Channels"() -> (w121:i32[])
                n114 = local read "Cmd"() -> (w119:T4[])
                n115 = for {
                  tunnel: w121 -> [w124] mode=indexing
                  shift-right: [w123] -> w118
                  shift-left: w119 -> [w125]
                  tunnel: w120 -> [w122]
                  n116 = in-place {
                    in-place-border: w122 -> [w126]
                    # "Index / Replace Array Element"
                    n117 = in-place-array #13(w125, w124) -> (w128:T4)
                    n118 = in-place {
                      in-place-border: w126 -> [w129]
                      n119 = in-place-cluster #14(w128) -> ()  [unwired: 1 out]
                      n120 = in-place-cluster #14("Digital Input"=w129) -> (w127:T4)
                    }
                    n121 = in-place-array #13(w127) -> (w123:T4[])  [unwired: 1 out]
                  }
                }
                n122 = property on="Cmd" class="Arr (strict)"("Val(Sgnl)"=w118) -> ()  [unwired: 2 in, 2 out]
              }
              frame #1 {
                n123 = property on="_Refresh" class="Bool (strict)"("Val(Sgnl)"=TRUE ("Value (Signaling)")) -> ()  [unwired: 2 in, 2 out]
              }
            }
          }
          event Value Change {
            n124 = event-data() -> ("NewVal"=w131:bool)  [unwired: 1 out]
            n125 = flat-sequence {
              tunnel: w131 -> [w134]
              frame #0 {
                n126 = local read "_HH Channels"() -> (w135:i32[])
                n127 = local read "Cmd"() -> (w133:T4[])
                n128 = for {
                  tunnel: w135 -> [w138] mode=indexing
                  shift-right: [w137] -> w132
                  shift-left: w133 -> [w139]
                  tunnel: w134 -> [w136]
                  n129 = in-place {
                    in-place-border: w136 -> [w140]
                    # "Index / Replace Array Element"
                    n130 = in-place-array #15(w139, w138) -> (w142:T4)
                    n131 = in-place {
                      in-place-border: w140 -> [w143]
                      n132 = in-place-cluster #16(w142) -> ()  [unwired: 1 out]
                      n133 = in-place-cluster #16("Polarity"=w143) -> (w141:T4)
                    }
                    n134 = in-place-array #15(w141) -> (w137:T4[])  [unwired: 1 out]
                  }
                }
                n135 = property on="Cmd" class="Arr (strict)"("Val(Sgnl)"=w132) -> ()  [unwired: 2 in, 2 out]
              }
              frame #1 {
                n136 = property on="_Refresh" class="Bool (strict)"("Val(Sgnl)"=TRUE ("Value (Signaling)")) -> ()  [unwired: 2 in, 2 out]
              }
            }
          }
          event Value Change {
            n137 = event-data() -> ("NewVal"=w145:sgl)  [unwired: 1 out]
            n138 = flat-sequence {
              tunnel: w145 -> [w148]
              frame #0 {
                n139 = local read "_HH Channels"() -> (w149:i32[])
                n140 = local read "Cmd"() -> (w147:T4[])
                n141 = for {
                  tunnel: w149 -> [w152] mode=indexing
                  shift-right: [w151] -> w146
                  shift-left: w147 -> [w153]
                  tunnel: w148 -> [w150]
                  n142 = in-place {
                    in-place-border: w150 -> [w154]
                    # "Index / Replace Array Element"
                    n143 = in-place-array #17(w153, w152) -> (w156:T4)
                    n144 = in-place {
                      in-place-border: w154 -> [w157]
                      n145 = in-place-cluster #18(w156) -> ()  [unwired: 1 out]
                      n146 = in-place-cluster #18("Frequency [Hz]"=w157) -> (w155:T4)
                    }
                    n147 = in-place-array #17(w155) -> (w151:T4[])  [unwired: 1 out]
                  }
                }
                n148 = property on="Cmd" class="Arr (strict)"("Val(Sgnl)"=w146) -> ()  [unwired: 2 in, 2 out]
              }
              frame #1 {
                n149 = property on="_Refresh" class="Bool (strict)"("Val(Sgnl)"=TRUE ("Value (Signaling)")) -> ()  [unwired: 2 in, 2 out]
              }
            }
          }
          event Value Change {
            n150 = event-data() -> ("NewVal"=w159:sgl)  [unwired: 1 out]
            n151 = flat-sequence {
              tunnel: w159 -> [w162]
              frame #0 {
                n152 = local read "_HH Channels"() -> (w163:i32[])
                n153 = local read "Cmd"() -> (w161:T4[])
                n154 = for {
                  tunnel: w163 -> [w166] mode=indexing
                  shift-right: [w165] -> w160
                  shift-left: w161 -> [w167]
                  tunnel: w162 -> [w164]
                  n155 = in-place {
                    in-place-border: w164 -> [w168]
                    # "Index / Replace Array Element"
                    n156 = in-place-array #19(w167, w166) -> (w170:T4)
                    n157 = in-place {
                      in-place-border: w168 -> [w171]
                      n158 = in-place-cluster #20(w170) -> ()  [unwired: 1 out]
                      n159 = in-place-cluster #20("Duty Cycle [%]"=w171) -> (w169:T4)
                    }
                    n160 = in-place-array #19(w169) -> (w165:T4[])  [unwired: 1 out]
                  }
                }
                n161 = property on="Cmd" class="Arr (strict)"("Val(Sgnl)"=w160) -> ()  [unwired: 2 in, 2 out]
              }
              frame #1 {
                n162 = property on="_Refresh" class="Bool (strict)"("Val(Sgnl)"=TRUE ("Value (Signaling)")) -> ()  [unwired: 2 in, 2 out]
              }
            }
          }
          event Value Change {
            n163 = event-data() -> ("NewVal"=w173:sgl)  [unwired: 1 out]
            n164 = flat-sequence {
              tunnel: w173 -> [w176]
              frame #0 {
                n165 = local read "_HH Channels"() -> (w177:i32[])
                n166 = local read "Cmd"() -> (w175:T4[])
                n167 = for {
                  tunnel: w177 -> [w180] mode=indexing
                  shift-right: [w179] -> w174
                  shift-left: w175 -> [w181]
                  tunnel: w176 -> [w178]
                  n168 = in-place {
                    in-place-border: w178 -> [w182]
                    # "Index / Replace Array Element"
                    n169 = in-place-array #21(w181, w180) -> (w184:T4)
                    n170 = in-place {
                      in-place-border: w182 -> [w185]
                      n171 = in-place-cluster #22(w184) -> ()  [unwired: 1 out]
                      n172 = in-place-cluster #22("TDC Offset [CAD]"=w185) -> (w183:T4)
                    }
                    n173 = in-place-array #21(w183) -> (w179:T4[])  [unwired: 1 out]
                  }
                }
                n174 = property on="Cmd" class="Arr (strict)"("Val(Sgnl)"=w174) -> ()  [unwired: 2 in, 2 out]
              }
              frame #1 {
                n175 = property on="_Refresh" class="Bool (strict)"("Val(Sgnl)"=TRUE ("Value (Signaling)")) -> ()  [unwired: 2 in, 2 out]
              }
            }
          }
          event Value Change {
            n176 = event-data() -> ("NewVal"=w187:sgl)  [unwired: 1 out]
            n177 = flat-sequence {
              tunnel: w187 -> [w190]
              frame #0 {
                n178 = local read "_HH Channels"() -> (w191:i32[])
                n179 = local read "Cmd"() -> (w189:T4[])
                n180 = for {
                  tunnel: w191 -> [w194] mode=indexing
                  shift-right: [w193] -> w188
                  shift-left: w189 -> [w195]
                  tunnel: w190 -> [w192]
                  n181 = in-place {
                    in-place-border: w192 -> [w196]
                    # "Index / Replace Array Element"
                    n182 = in-place-array #23(w195, w194) -> (w198:T4)
                    n183 = in-place {
                      in-place-border: w196 -> [w199]
                      n184 = in-place-cluster #24(w198) -> ()  [unwired: 1 out]
                      n185 = in-place-cluster #24("Window Start [DBTDC]"=w199) -> (w197:T4)
                    }
                    n186 = in-place-array #23(w197) -> (w193:T4[])  [unwired: 1 out]
                  }
                }
                n187 = property on="Cmd" class="Arr (strict)"("Val(Sgnl)"=w188) -> ()  [unwired: 2 in, 2 out]
              }
              frame #1 {
                n188 = property on="_Refresh" class="Bool (strict)"("Val(Sgnl)"=TRUE ("Value (Signaling)")) -> ()  [unwired: 2 in, 2 out]
              }
            }
          }
          event Value Change {
            n189 = event-data() -> ("NewVal"=w201:sgl)  [unwired: 1 out]
            n190 = flat-sequence {
              tunnel: w201 -> [w204]
              frame #0 {
                n191 = local read "_HH Channels"() -> (w205:i32[])
                n192 = local read "Cmd"() -> (w203:T4[])
                n193 = for {
                  tunnel: w205 -> [w208] mode=indexing
                  shift-right: [w207] -> w202
                  shift-left: w203 -> [w209]
                  tunnel: w204 -> [w206]
                  n194 = in-place {
                    in-place-border: w206 -> [w210]
                    # "Index / Replace Array Element"
                    n195 = in-place-array #25(w209, w208) -> (w212:T4)
                    n196 = in-place {
                      in-place-border: w210 -> [w213]
                      n197 = in-place-cluster #26(w212) -> ()  [unwired: 1 out]
                      n198 = in-place-cluster #26("Window End [DBTDC]"=w213) -> (w211:T4)
                    }
                    n199 = in-place-array #25(w211) -> (w207:T4[])  [unwired: 1 out]
                  }
                }
                n200 = property on="Cmd" class="Arr (strict)"("Val(Sgnl)"=w202) -> ()  [unwired: 2 in, 2 out]
              }
              frame #1 {
                n201 = property on="_Refresh" class="Bool (strict)"("Val(Sgnl)"=TRUE ("Value (Signaling)")) -> ()  [unwired: 2 in, 2 out]
              }
            }
          }
          event Value Change {
            n202 = event-data() -> ("NewVal"=w215:T7[])  [unwired: 1 out]
            n203 = flat-sequence {
              tunnel: w215 -> [w218]
              frame #0 {
                n204 = local read "_HH Channels"() -> (w219:i32[])
                n205 = local read "Cmd"() -> (w217:T4[])
                n206 = for {
                  tunnel: w219 -> [w222] mode=indexing
                  shift-right: [w221] -> w216
                  shift-left: w217 -> [w223]
                  tunnel: w218 -> [w220]
                  n207 = in-place {
                    in-place-border: w220 -> [w224]
                    # "Index / Replace Array Element"
                    n208 = in-place-array #27(w223, w222) -> (w226:T4)
                    n209 = in-place {
                      in-place-border: w224 -> [w228]
                      n210 = in-place-cluster #28(w226) -> ()  [unwired: 1 out]
                      n211 = Reshape Array(w228, 4 ("dimension size")) -> (w227:T7[])
                      n212 = in-place-cluster #28("Angles"=w227) -> (w225:T4)
                    }
                    n213 = in-place-array #27(w225) -> (w221:T4[])  [unwired: 1 out]
                  }
                }
                n214 = property on="Cmd" class="Arr (strict)"("Val(Sgnl)"=w216) -> ()  [unwired: 2 in, 2 out]
              }
              frame #1 {
                n215 = property on="_Refresh" class="Bool (strict)"("Val(Sgnl)"=TRUE ("Value (Signaling)")) -> ()  [unwired: 2 in, 2 out]
              }
            }
          }
          event Value Change {
            n216 = event-data() -> ("NewVal"=w231:bool)  [unwired: 1 out]
            n217 = flat-sequence {
              tunnel: w231 -> [w234]
              frame #0 {
                n218 = local read "_HH Channels"() -> (w235:i32[])
                n219 = local read "Cmd"() -> (w233:T4[])
                n220 = for {
                  tunnel: w235 -> [w238] mode=indexing
                  shift-right: [w237] -> w232
                  shift-left: w233 -> [w239]
                  tunnel: w234 -> [w236]
                  n221 = in-place {
                    in-place-border: w236 -> [w240]
                    # "Index / Replace Array Element"
                    n222 = in-place-array #29(w239, w238) -> (w242:T4)
                    n223 = in-place {
                      in-place-border: w240 -> [w243]
                      n224 = in-place-cluster #30(w242) -> ()  [unwired: 1 out]
                      n225 = in-place-cluster #30("Skip Fire"=w243) -> (w241:T4)
                    }
                    n226 = in-place-array #29(w241) -> (w237:T4[])  [unwired: 1 out]
                  }
                }
                n227 = property on="Cmd" class="Arr (strict)"("Val(Sgnl)"=w232) -> ()  [unwired: 2 in, 2 out]
              }
              frame #1 {
                n228 = property on="_Refresh" class="Bool (strict)"("Val(Sgnl)"=TRUE ("Value (Signaling)")) -> ()  [unwired: 2 in, 2 out]
              }
            }
          }
          event Value Change {
            n229 = event-data() -> ("NewVal"=w245:u8)  [unwired: 1 out]
            n230 = flat-sequence {
              tunnel: w245 -> [w248]
              frame #0 {
                n231 = local read "_HH Channels"() -> (w249:i32[])
                n232 = local read "Cmd"() -> (w247:T4[])
                n233 = for {
                  tunnel: w249 -> [w252] mode=indexing
                  shift-right: [w251] -> w246
                  shift-left: w247 -> [w253]
                  tunnel: w248 -> [w250]
                  n234 = in-place {
                    in-place-border: w250 -> [w254]
                    # "Index / Replace Array Element"
                    n235 = in-place-array #31(w253, w252) -> (w256:T4)
                    n236 = in-place {
                      in-place-border: w254 -> [w257]
                      n237 = in-place-cluster #32(w256) -> ()  [unwired: 1 out]
                      n238 = in-place-cluster #32("Skip Fire Index"=w257) -> (w255:T4)
                    }
                    n239 = in-place-array #31(w255) -> (w251:T4[])  [unwired: 1 out]
                  }
                }
                n240 = property on="Cmd" class="Arr (strict)"("Val(Sgnl)"=w246) -> ()  [unwired: 2 in, 2 out]
              }
              frame #1 {
                n241 = property on="_Refresh" class="Bool (strict)"("Val(Sgnl)"=TRUE ("Value (Signaling)")) -> ()  [unwired: 2 in, 2 out]
              }
            }
          }
          event "_AdaptMode": Value Change {
            n242 = event-data() -> ()  [unwired: 7 out]
            n243 = local read "_HH Channels"() -> (w263:i32[])
            n244 = Number To Boolean Array(number="AdaptMode") -> (Boolean array=w261:bool[])
            n245 = for {
              tunnel: "_AdaptMode" -> [w272]
              shift-right: [w270] -> w260
              shift-left: w261 -> [w269]
              tunnel: w263 -> [w271] mode=indexing
              n246 = Replace Array Subset(array=w269, new element=w272, index=w271) -> (w270:bool[])
            }
            n247 = Select(t=T10."Disabled and Grayed Out" ("Disabled"), s="_AdaptMode", f=T10."Enabled" ("Disabled")) -> (s? t:f=w264:T10)
            n248 = Boolean Array To Number(Boolean array=w260) -> (number=w259:u32)
            n249 = property on="_Command" class="Clust (strict)"("DisabledEnum"=w264) -> ()  [unwired: 2 in, 2 out]
            n250 = property on="AdaptMode" class="DigNum (strict)"("Val(Sgnl)"=w259) -> ()  [unwired: 2 in, 2 out]
            n251 = property on="_Refresh" class="Bool (strict)"("Val(Sgnl)"=TRUE ("Value (Signaling)")) -> ()  [unwired: 2 in, 2 out]
          }
          event "_HH Channels": Value Change {
            n252 = event-data() -> ()  [unwired: 2 out]
            n253 = property on="_Refresh" class="Bool (strict)"("Val(Sgnl)"=TRUE ("Value (Signaling)")) -> ()  [unwired: 2 in, 2 out]
          }
          event "_Refresh": Value Change {
            n254 = event-data() -> ()  [unwired: 2 out]
            n255 = local write "_Refresh"(FALSE ("_Refresh")) -> ()
            n256 = stacked-sequence {
              frame #0 {
                n257 = local read "ChannelNames"() -> (w276:string[])
                n258 = local read "_HH Channels"() -> (w289:i32[])
                n259 = local read "AdaptMode"() -> (w285:u32)
                n260 = local read "Config"() -> (w286:T1)
                n261 = local read "Cmd"() -> (w287:T4[])
                n262 = Index Array(array=w289, index=0) -> (element=w275:i32)
                n263 = Number To Boolean Array(number=w285) -> (Boolean array=w288:bool[])
                n264 = Index Array(array=w286, index=w275) -> (element=w280:T9)
                n265 = Index Array(array=w287, index=w275) -> (element=w279:T4)
                n266 = Index Array(array=w276, index=w275) -> (element=w278:string)
                n267 = Index Array(array=w288, index=w275) -> (element=w277:bool)
                n268 = Select(t=T10."Disabled and Grayed Out" ("Disabled"), s=w277, f=T10."Enabled" ("Disabled")) -> (s? t:f=w283:T10)
                n269 = local write "_AdaptMode"(w277) -> ()
                n270 = local write "_Config Element"(w280) -> ()
                n271 = local write "_Command Element"(w279) -> ()
                n272 = local write "_Channel Name"(w278) -> ()
                n273 = property on="_Command" class="Clust (strict)"("DisabledEnum"=w283) -> ()  [unwired: 2 in, 2 out]
              }
              frame #1 {
                n274 = local read "_Config Element"() -> (w296:T9)
                n275 = control-ref of="_Command Element"() -> (w291:refnum<vi>)
                n276 = control-ref of="_Listbox"() -> (w292:refnum<vi>)
                n277 = local read "ChannelNames"() -> (w290:string[])
                n278 = Unbundle By Name(w296) -> ("Mode"=w295:T2)
                n279 = call "HH Command Disable.vi"("_Command"=w291) -> ()  [unwired: 11 in]
                n280 = local read "AdaptMode"() -> (w299:u32)
                n281 = local read "Config"() -> (w301:T1)
                n282 = local read "Cmd"() -> (w300:T4[])
                n283 = To Unsigned Long Integer(number=w295) -> (unsigned 32bit integer=w294:u32)
                n284 = call "Refresh HH Listbox.vi"("AdaptMode"=w299, "Command"=w300, "Names"=w290, "Config"=w301, "_Listbox"=w292) -> ("Config out"=w293:T11[], "AdaptMode"=w298:u32, "Disabled Configs"=→"_Disabled Configs":i32[])  [unwired: 3 in, 1 out]
                n285 = local write "_Icon tabs"(w294) -> ()
                n286 = property on="AdaptMode" class="DigNum (strict)"("Val(Sgnl)"=w298) -> ()  [unwired: 2 in, 2 out]
                n287 = local write "Config"(w293) -> ()
              }
            }
          }
        }
      }
    }
  }
